vi "configure.vi"(8 "error in (no error)":errorcluster, 9 "Value":i32, 10 "ILC":refnum<class "ILC.lvclass">, 11 "ConfigureILCMotorDriveStrategy in":refnum<class "ConfigureILCMotorDriveStrategy.lvclass">) -> (0 "error out":errorcluster, 3 "ConfigureILCMotorDriveStrategy out":refnum<class "ConfigureILCMotorDriveStrategy.lvclass">)   [LabVIEW 2015, in "ConfigureILCMotorDriveStrategy.lvclass"]
uses:
  ConfigureILCMotorDriveStrategy.lvclass
  <userlib>/Common/ILC/ILC/ILC.lvclass
  ConfigureILCMotorDriveStrategy.lvclass/ConfigureILCMotorDriveStrategy.ctl
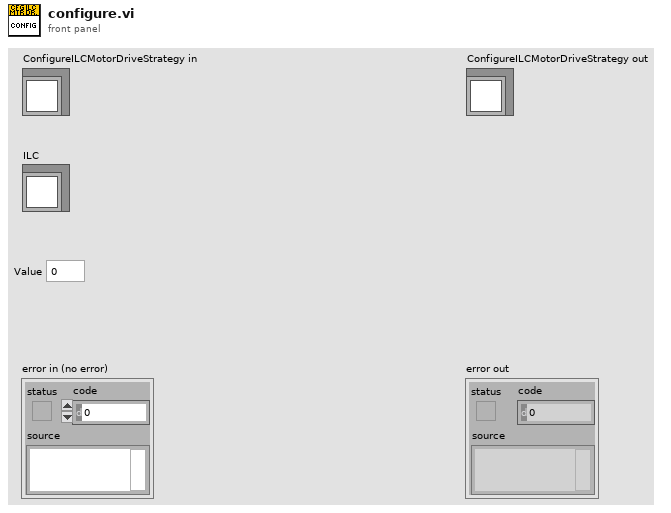
[diagram p1: front panel]
types:
  T1 = typedef "ILCBTTypedefs.lvlib/MUX Signals.ctl" = cluster{"MUX_A0 DAQ Channel to Write":refnum<k21>, "MUX_A1 DAQ Channel to Write":refnum<k21>}
  T2 = typedef "ILCBTTypedefs.lvlib/MUX Settings.ctl" = cluster{"MUX_AO":T3, "MUX_A1":T3}
  T3 = typedef "ILCBTTypedefs.lvlib/Digital Signal Level.ctl" = enum16{"Low", "High"}
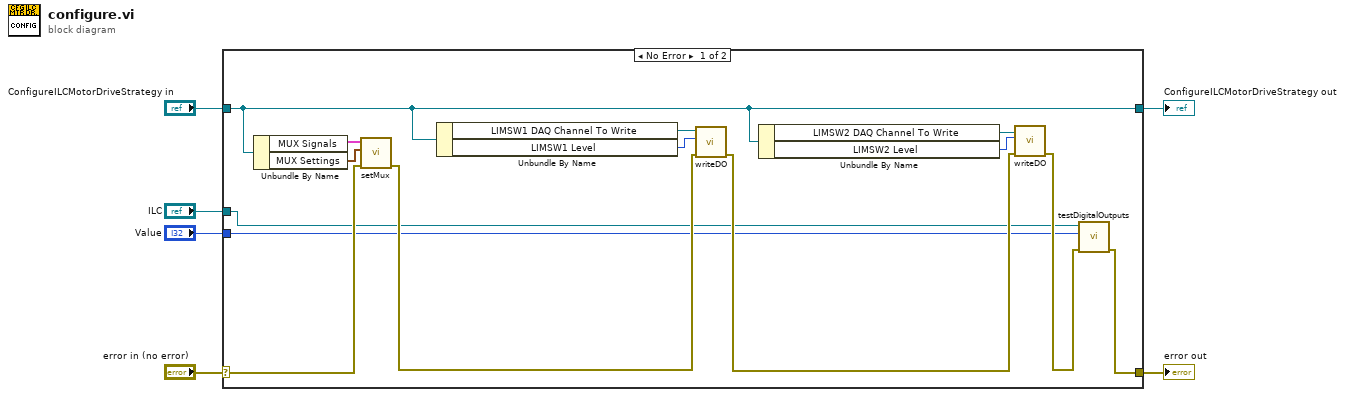
[diagram p0: block diagram]
diagram:
  n1 = case shown="No Error" "error in (no error)" {
    selector: "error in (no error)" -> [w19 w22]
    tunnel: [w18 w22] -> w5
    tunnel: [w16 w21] -> w3
    tunnel: "ConfigureILCMotorDriveStrategy in" -> [w16 w21]
    tunnel: "ILC" -> [w9 _]
    tunnel: "Value" -> [w8 _]
    frame No Error {
      n2 = Unbundle By Name(w16) -> ("MUX Signals"=w20:T1, "MUX Settings"=w7:T2)
      n3 = call "setMux.vi"("error in (no error)"=w19, "MUX Settings"=w7, "MUX Signals"=w20) -> ("error out"=w10:errorcluster)  [unwired: 8 in]
      n4 = Unbundle By Name(w16) -> ("LIMSW1 DAQ Channel To Write"=w15:refnum<k21>, "LIMSW1 Level"=w17:T3)
      n5 = call "writeDO.vi"("error in"=w10, "Digital Signal Level"=w17, "DAQmx Global Channel"=w15) -> ("error out"=w12:errorcluster)  [unwired: 8 in]
      n6 = Unbundle By Name(w16) -> ("LIMSW2 DAQ Channel To Write"=w14:refnum<k21>, "LIMSW2 Level"=w13:T3)
      n7 = call "writeDO.vi"("error in"=w12, "Digital Signal Level"=w13, "DAQmx Global Channel"=w14) -> ("error out"=w11:errorcluster)  [unwired: 8 in]
      n8 = call <userlib>:"testDigitalOutputs.vi"("error in (no error)"=w11, "Digital Output Value"=w8, "ILC in"=w9) -> ("error out"=w18:errorcluster)  [unwired: 7 in, 1 out]
    }
    frame Error {
    }
  }
  "error out" <- w5
  "ConfigureILCMotorDriveStrategy out" <- w3
